vi "timing.vi"(11 "Feedback loop time":u32=5) -> (3 "Feedback Loop time":u32)   [LabVIEW 2019]
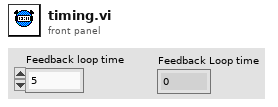
[diagram p1: front panel]
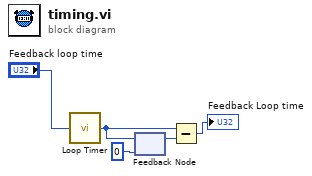
[diagram p0: block diagram]
diagram:
  n1 = call "Loop Timer"("Count(uSec)"="Feedback loop time") -> ("Tick Count(uSec)"=w2:u32)
  n2 = feedback #1(u32 0 ("Tick Count(uSec)")) -> (w3:u32)
  n3 = feedback-in #1(w2) -> ()
  n4 = Subtract(x=w2, y=w3) -> (x-y=→"Feedback Loop time":u32)
